vi "PIM Manage Strip Chart Display.vi"(7 "Clear?":bool, 10 "IM Power(s)":dbl[](array[numeric]), 11 "PIM Test Parameters":T1={"Stimulus"={"C1 Pwr dBm"=0.0, "C2 Pwr dBm"=0.0, "Power Units"=enum."dBm", "Meas Type"=enum."Time", "C1 Freq MHz"=0.0, "C2 Freq MHz"=0.0, "Swept Freq Step"=0}, "Measure"={"IM Order"=0, "Direction"=0, "Averaging"=1, "ALC ON?"=TRUE, "Peak Hold?"=TRUE, "Peak last N"=1, "Ref Level dBm"=-100.0, "Ref Units"=enum."dBm", "Num Samples"=1, "Sample units"=enum."Sample(s)", "Update Rate (s)"=0.0, "DUT PORT"=enum."Port 1", "Percent (%)"=100}, "Display"={"Power Scale"={"yRange_min"=0, "yRange_max"=0}, "xRange_span"=5}} {"Stimulus"."Swept Freq Step" items=[".2", ".4", "1.0", "2.0"]; "Measure"."Averaging" items=["None", "Minimum", "Normal", "High", "Maximum"]; "Measure"."Direction" items=["Reverse", "Forward", "Auxiliary"]; "Measure"."IM Order" items=["3rd", "5th", "7th", "9th", "11th", "13th", "15th", "17th", "19th", "21st", "23rd", "25th", "27th", "29th", "31st", "33rd"]}) -> (1 "Strip Total Span (seconds|samples)":dbl, 2 "Strip Window Span (seconds|samples)":dbl, 3 "PIM Traces":cluster{"x-values":dbl[], "y-values":dbl[]}[](array[cluster]), 5 "Point Plotted?":bool)   [LabVIEW 2011]
uses:
  TypeDefs/PIM Test Parameters.ctl
  TypeDefs/PIM Stimulus Parameters.ctl
  SI.LIB/PIM.LIB/HW IO/PIM Sweep Step Size.ctl
  TypeDefs/PIM Measurement Parameters.ctl
  SI.LIB/PIM.LIB/HW IO/IMOrder.ctl
  SI.LIB/PIM.LIB/HW IO/MeasMode.ctl
  SI.LIB/PIM.LIB/HW IO/HW Averaging.ctl
  TypeDefs/PIM Meas Units.ctl
  SI.LIB/PIM.LIB/HW IO/DUTport.ctl
  TypeDefs/PIM Display Parameters.ctl
  SI.LIB/PIM.LIB/DISPLAY/Strip Chart Display Data.ctl
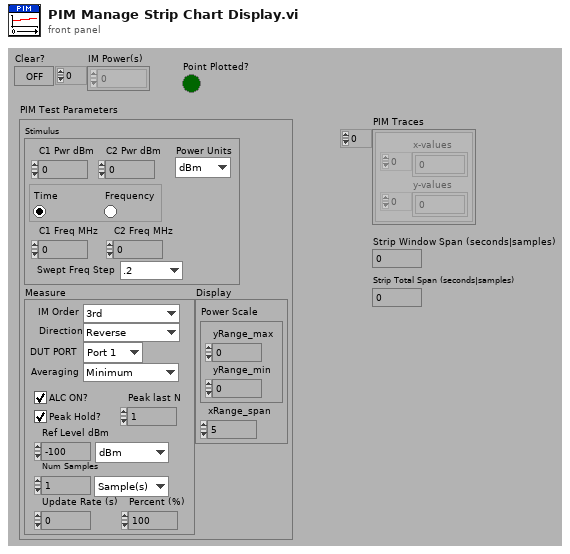
[diagram p1: front panel]
types:
  T1 = typedef "PIM Test Parameters.ctl" = cluster{"Stimulus":T2, "Measure":T4, "Display":T10}
  T2 = typedef "PIM Stimulus Parameters.ctl" = cluster{"C1 Pwr dBm":dbl, "C2 Pwr dBm":dbl, "Power Units":enum16{"dBm", "Watts"}, "Meas Type":enum32{"Time", "Frequency"}, "C1 Freq MHz":dbl, "C2 Freq MHz":dbl, "Swept Freq Step":T3}
  T3 = typedef "PIM Sweep Step Size.ctl" = u16
  T4 = typedef "PIM Measurement Parameters.ctl" = cluster{"IM Order":T5, "Direction":T6, "Averaging":T7, "ALC ON?":bool, "Peak Hold?":bool, "Peak last N":u32, "Ref Level dBm":dbl, "Ref Units":enum16{"dBm", "dBc"}, "Num Samples":u32, "Sample units":T8, "Update Rate (s)":dbl, "DUT PORT":T9, "Percent (%)":u8}
  T5 = typedef "IMOrder.ctl" = u8
  T6 = typedef "MeasMode.ctl" = u16
  T7 = typedef "HW Averaging.ctl" = u16
  T8 = typedef "PIM Meas Units.ctl" = enum16{"Sample(s)", "Second(s)", "Sweep(s)"}
  T9 = typedef "DUTport.ctl" = enum16{"Port 1", "Port 2"}
  T10 = typedef "PIM Display Parameters.ctl" = cluster{"Power Scale":cluster{"yRange_min":i32, "yRange_max":i32}, "xRange_span":u32}
  T11 = typedef "Strip Chart Display Data.ctl" = cluster{"Reference Value":dbl, "Update Rate (s)":dbl, "Time Scale":dbl, "Hold":bool, "Clear":bool, "History Windows":i32, "HistoryView":bool}
  T12 = typedef "PIM Stimulus.ctl" = cluster{"Carrier Frequencies":cluster{"C1 Freq, MHz":dbl, "C2 Freq, MHz":dbl}, "Carrier Powers":cluster{"C1 Power,dBm":dbl, "C2 Power, dBm":dbl}, "Measurement Parameters":T13, "Measurement Setup":cluster{"Meas Type":enum32{"Time", "Frequency"}, "TXStep":T3}}
  T13 = typedef "PIM Cmd Params.ctl" = cluster{"IM Order":T5, "Averaging":T7, "Direction":T6, "Enable ALC?":bool, "Enable SingleIM?":bool, "Display Units":T14, "VA Hold?":bool, "DUT PORT":T9}
  T14 = typedef "display_unit_format.ctl" = enum16{"dBm", "dBc"}
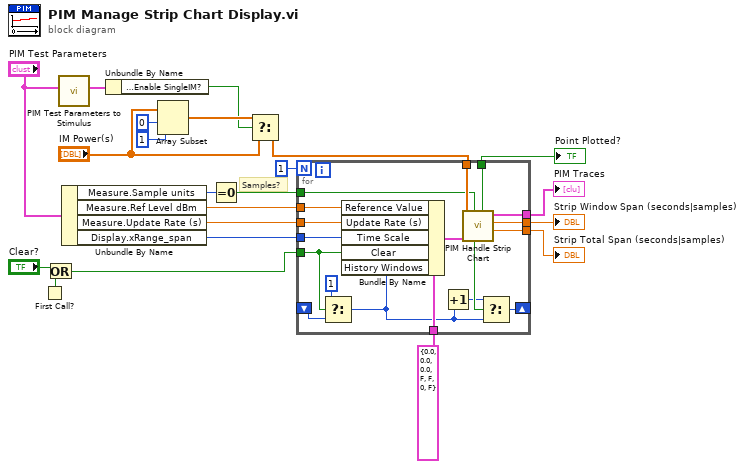
[diagram p0: block diagram]
diagram:
  # "Samples?"
  n1 = First Call?() -> (First Call?: T/F=w21:bool)
  n2 = Or(x="Clear?", y=w21) -> (x .or. y?=w19:bool)
  n3 = call "PIM Test Parameters to Stimulus.vi"("PIM Test Parameters"="PIM Test Parameters") -> ("PIM Measurement Stimulus"=w8:T12)  [unwired: 10 out]
  n4 = Unbundle By Name("PIM Test Parameters") -> ("Measure.Sample units"=w13:T8, "Measure.Ref Level dBm"=w14:dbl, "Measure.Update Rate (s)"=w11:dbl, "Display.xRange_span"=w15:u32)
  n5 = Unbundle By Name(w8) -> ("Measurement Parameters.Enable SingleIM?"=w4:bool)
  n6 = Array Subset(array="IM Power(s)", index=0, length=1) -> (w5:dbl[])
  n7 = Equal To 0?(x=w13) -> (x = 0?=w12:bool)
  n8 = Select(t=w5, s=w4, f="IM Power(s)") -> (s? t:f=w2:dbl[])
  n9 = for {
    N: 1 -> [_]
    tunnel: T11 {"Reference Value"=0.0, "Update Rate (s)"=0.0, "Time Scale"=0.0, "Hold"=FALSE, "Clear"=FALSE, "History Windows"=0, "HistoryView"=FALSE} ("Strip Chart Display Data") -> [w40]
    tunnel: w15 -> [w39]
    tunnel: w2 -> [w38]
    tunnel: w19 -> [w34]
    tunnel: [w36] -> w1
    shift-right: [w29] -> _
    shift-left: _ -> [w33]
    tunnel: [w28] -> w18
    tunnel: [w27] -> w17
    tunnel: w14 -> [w26]
    tunnel: w12 -> [w25]
    tunnel: w11 -> [w24]
    tunnel: [w23] -> w10
    n10 = Select(t=1 ("Update Rate"), s=w34, f=w33) -> (s? t:f=w30:i32)
    n11 = Bundle By Name(cluster=w40, "Reference Value"=w26, "Update Rate (s)"=w24, "Time Scale"=w39, "Clear"=w34, "History Windows"=w30) -> (w37:T11)
    n12 = Increment(x=w30) -> (x+1=w31:i32)
    n13 = call "PIM Handle Strip Chart.vi"("Strip by sample? (F = seconds)"=w25, "Strip Chart Display Data"=w37, "Measured PIM (dBm/dBc)"=w38) -> ("Strip Total Span (seconds|samples)"=w27:dbl, "Strip Window Span (seconds|samples)"=w28:dbl, "PIM Traces"=w36:cluster{"x-values":dbl[], "y-values":dbl[]}[], "Point Plotted?"=w23:bool, "Increment History?"=w32:bool)  [unwired: 4 out]
    n14 = Select(t=w31, s=w32, f=w30) -> (s? t:f=w29:i32)
  }
  "PIM Traces" <- w1
  "Strip Window Span (seconds|samples)" <- w18
  "Strip Total Span (seconds|samples)" <- w17
  "Point Plotted?" <- w10
